vi "Write To Spreadsheet File_extended.vi"(0 "delimiter (Tab)":string="\t", 1 "transpose? (no:F)":bool, 4 "format (%.3f)":string="%.3f", 5 "header":string, 6 "append to file? (new file:F)":bool, 7 "1D data":dbl[](array[numeric]) format="%.2f", 9 "2D data":dbl[][](array[numeric]) format="%.2f", 10 "file path (dialog if empty)":path) -> (3 "new file path (Not A Path if cancelled)":path)   [LabVIEW 2013]
doc: "Converts a 2D or 1D array of single-precision (SGL) numbers to a text string and writes the string to a new byte stream file or appends the string to an existing file."
panel:
  out "error out":errorcluster
  in  "prompt":string="Choose file to write."
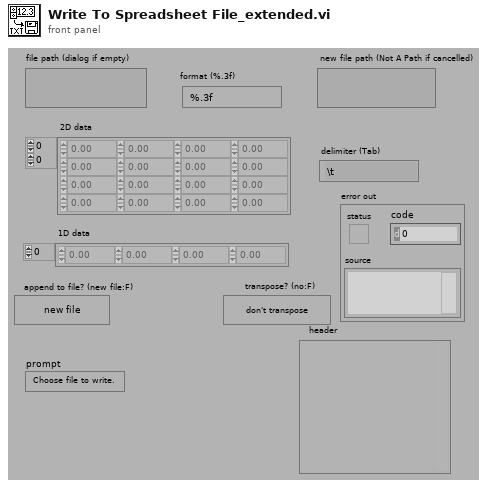
[diagram p1: front panel]
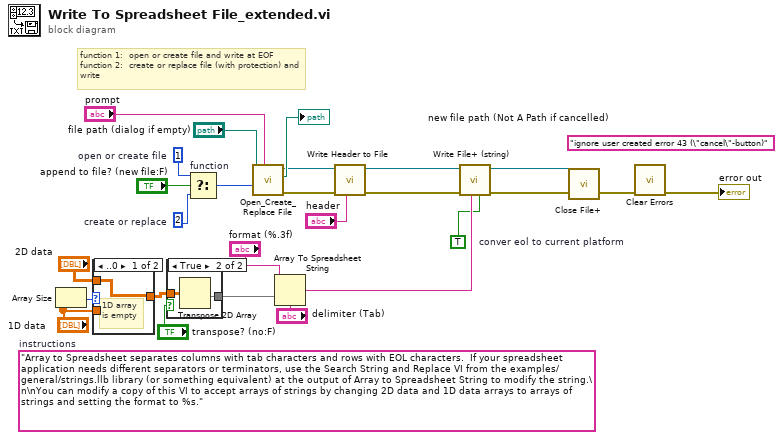
[diagram p0: block diagram]
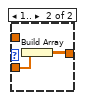
[diagram p3: hidden frame]
diagram:
  (unwired) "ignore user created error 43 (\"cancel\"-button)"
  (unwired) "Array to Spreadsheet separates columns with tab characters and rows with EOL characters.  If your spreadsheet application needs different separators or terminators, use the Search String and Replace VI from the examples/general/strings.llb library (or something equivalent) at the output of Array to Spreadsheet String to modify the string.\n\nYou can modify a copy of this VI to accept arrays of strings by changing 2D data and 1D data arrays to arrays of strings and setting the format to %s."  # instructions
  w11 = i16 2  # create or replace
  w8 = TRUE  # conver eol to current platform
  w24 = i16 1  # open or create file
  # "function 1:  open or create file and write at EOF\nfunction 2:  create or replace file (with protection) and write"
  n1 = Array Size(array="1D data") -> (size(s)=w23:i32)
  n2 = case shown="..0" w23 {
    tunnel: "1D data" -> [_ w28]
    tunnel: [w26 w27] -> w19
    tunnel: "2D data" -> [w26 _]
    frame ..0 {
      # "1D array is empty"
    }
    frame 1.. {
      n3 = Build Array(w28) -> (w27:dbl[][])
    }
  }
  n4 = case shown="True" "transpose? (no:F)" {
    tunnel: [w29 w31] -> w17
    tunnel: w19 -> [w29 w30]
    frame False {
    }
    frame True {
      n5 = Transpose 2D Array(2D array=w30) -> (transposed array=w31:dbl[][])
    }
  }
  n6 = Select "function"(t=w24, s="append to file? (new file:F)", f=w11) -> (s? t:f=w16:i16)
  n7 = call <vilib>:"Open_Create_Replace File.vi"("prompt"="prompt", "function (open:0)"=w16, "file path"="file path (dialog if empty)") -> ("error out"=w7:errorcluster, "new file path"=→"new file path (Not A Path if cancelled)":path, "refnum"=w2:refnum<file>)  [unwired: 5 in, 1 out]
  n8 = Array To Spreadsheet String(delimiter (Tab)="delimiter (Tab)", array=w17, 3:"format (%.3f)") -> (spreadsheet string=w14:string)
  n9 = call "Write Header to File"("string"="header", "refnum"=w2) -> ("dup refnum"=w1:refnum<file>)  [unwired: 5 in, 2 out]
  n10 = call <vilib>:"Write File+ (string).vi"("convert eol? (no:F)"=w8, "string"=w14, "error in (no error)"=w7, "refnum"=w1) -> ("error out"=w6:errorcluster, "dup refnum"=w13:refnum<file>)  [unwired: 3 in, 1 out]
  n11 = call <vilib>:"Close File+.vi"("error in (no error)"=w6, "refnum"=w13) -> ("error out"=w5:errorcluster)  [unwired: 3 in, 2 out]
  n12 = call <vilib>:"Clear Errors.vi"("error in (no error)"=w5) -> ("error out"=→"error out":errorcluster)  [unwired: 6 in]
